vi "parseQuery.vi"(8 "error in (no error)":errorcluster, 10 "QueryString":string, 11 "CommandParser in":refnum<class "CommandParser.lvclass">) -> (0 "error out":errorcluster, 2 "MonoCommand":T1, 3 "CommandParser out":refnum<class "CommandParser.lvclass">)   [LabVIEW 2016, in "CommandParser.lvclass"]
uses:
  CommandParser.lvclass
  Typedefs/MonoCommand.ctl
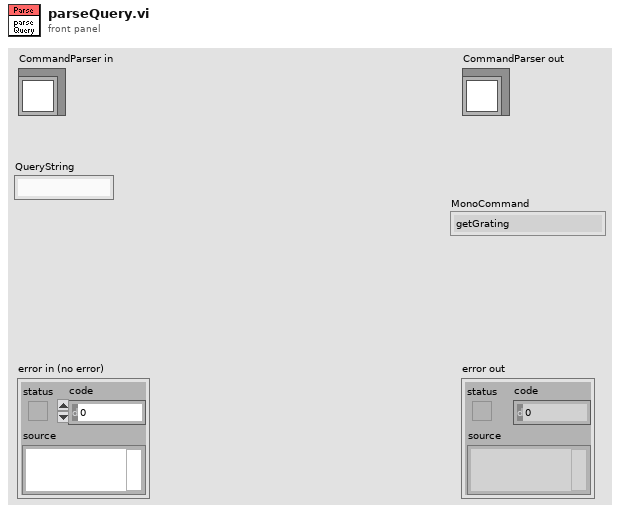
[diagram p1: front panel]
types:
  T1 = typedef "MonoCommand.ctl" = enum16{"getGrating", "getFrontEntranceSlitPosition", "getFrontExitSlitPosition", "getWavelength", "setWavelength", "setGrating", "setFrontEntranceSlitPosition", "setFrontExitSlitPosition", "calibrateWavelength", "getStatus", "Unknown", "reset"}
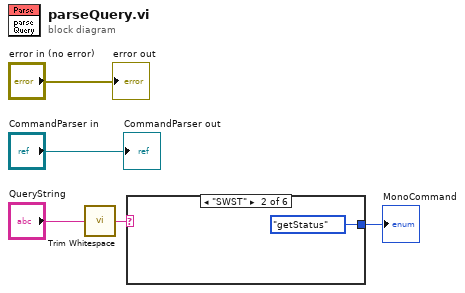
[diagram p0: block diagram]
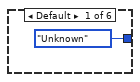
[diagram p2: hidden frame]
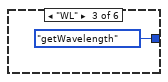
[diagram p3: hidden frame]
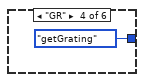
[diagram p4: hidden frame]
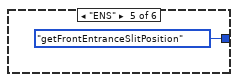
[diagram p5: hidden frame]
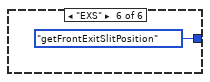
[diagram p6: hidden frame]
diagram:
  n1 = call <vilib>:"Trim Whitespace.vi"("string"="QueryString") -> ("trimmed string"=w1:string)  [unwired: 1 in]
  n2 = case shown="\"SWST\"" w1 {
    tunnel: [MonoCommand."Unknown" ("MonoCommand") MonoCommand."getStatus" ("MonoCommand") MonoCommand."getWavelength" ("MonoCommand") MonoCommand."getGrating" ("MonoCommand") MonoCommand."getFrontEntranceSlitPosition" ("MonoCommand") MonoCommand."getFrontExitSlitPosition" ("MonoCommand")] -> w3
    frame Default {
    }
    frame "SWST" {
    }
    frame "WL" {
    }
    frame "GR" {
    }
    frame "ENS" {
    }
    frame "EXS" {
    }
  }
  "MonoCommand" <- w3
  "error out" <- "error in (no error)"
  "CommandParser out" <- "CommandParser in"
